vi "Config.Lookup Name from Variant Attr List.vi"(10 "Name In":string, 11 "Variant":variant) -> (2 "Name Out":string)   [LabVIEW 2018]
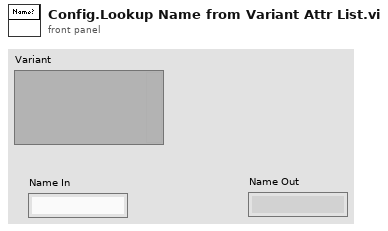
[diagram p1: front panel]
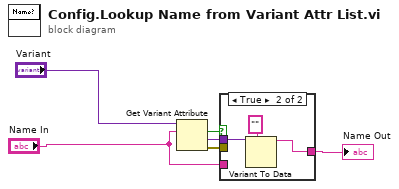
[diagram p0: block diagram]
diagram:
  n1 = Get Variant Attribute(Variant="Variant", name="Name In") -> (found=w6:bool, value=w5:variant, error out=w4:errorcluster)  [unwired: 2 in, 1 out]
  n2 = case shown="True" w6 {
    tunnel: w5 -> [_ w10]
    tunnel: w4 -> [_ _]
    tunnel: [w7 w8] -> w1
    tunnel: "Name In" -> [w7 _]
    frame False {
    }
    frame True {
      n3 = Variant To Data(type="", Variant=w10) -> (data=w8:string)  [unwired: 1 in, 1 out]
    }
  }
  "Name Out" <- w1
